vi "GenerateWebSocketClientKey.vi"() -> (3 "WebSocket Key":string)   [LabVIEW 2013, in "WebSockets.lvlib"]
doc: "Generates a random string of 16 ASCII characters (from ASCII 37 to 127) for the Sec-WebSocket-Key."
uses:
  WebSockets.lvlib
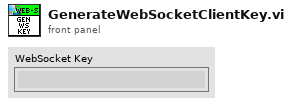
[diagram p1: front panel]
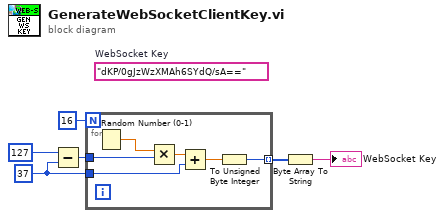
[diagram p0: block diagram]
diagram:
  w2 = u8 37 ("lower limit")
  (unwired) "dKP/0gJzWzXMAh6SYdQ/sA=="  # WebSocket Key
  n1 = Subtract(x=u8 127 ("upper limit"), y=w2) -> (x-y=w1:u8)
  n2 = for {
    N: 16 -> [_]
    tunnel: [w8] -> w5 mode=indexing
    tunnel: w2 -> [w11]
    tunnel: w1 -> [w10]
    n3 = Random Number (0-1)() -> (number: 0 to 1=w7:dbl)
    n4 = Multiply(x=w7, y=w10) -> (x*y=w12:dbl)
    n5 = Add(x=w12, y=w11) -> (x+y=w9:dbl)
    n6 = To Unsigned Byte Integer(number=w9) -> (unsigned 8bit integer=w8:u8)
  }
  n7 = Byte Array To String(unsigned byte array=w5) -> (string=→"WebSocket Key":string)
